vi "tcs_getSample_Timestamp.vi"(8 "error in (no error)":errorcluster, 11 "Timestamp_Ctl":T1) -> (0 "error out":errorcluster, 2 "function return":i32, 3 "Timestamp_Ctl out":T1)   [LabVIEW 2016, in "SALLV_tcs.lvlib"]
doc: "int tcs_shm_getSample_TimestampLV(tcs_TimestampLV *Timestamp_Ctl );"
uses:
  SALLV_tcs.lvlib
  DataTypes/Timestamp.ctl
  SALLV_tcs.so
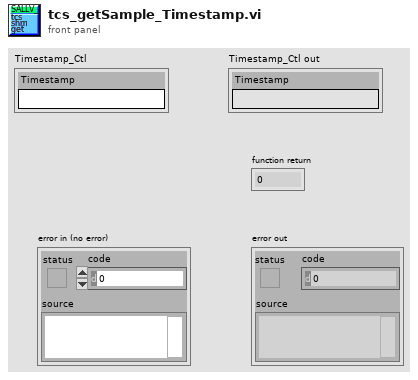
[diagram p1: front panel]
types:
  T1 = typedef "SALLV_tcs.lvlib/Timestamp.ctl" = cluster{"Timestamp":string}
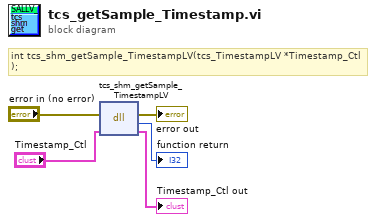
[diagram p0: block diagram]
diagram:
  # "int tcs_shm_getSample_TimestampLV(tcs_TimestampLV *Timestamp_Ctl );"
  n1 = dll-call lib="home/saluser/ct_tcs/ts_sallv_tcs/SALLV_tcs.*" fn="tcs_shm_getSample_TimestampLV"(error in="error in (no error)", "Timestamp_Ctl"="Timestamp_Ctl") -> (error out=→"error out":errorcluster, →"function return":i32, "Timestamp_Ctl"=→"Timestamp_Ctl out":T1)  [unwired: 2 in, 1 out]
